vi "RTS Rebuild Custom Array.vi"(8 "Error In":errorcluster, 9 "Index Locations":i32[](array[numeric]), 10 "Full Item Names":string[](array[string]), 11 "File Location":path) -> (0 "Error Out":errorcluster, 3 "Correctly Indexed Array":dbl[][](array[numeric]))   [LabVIEW 2020]
panel:
  out "size(s) 2":i32[](array[numeric])
  out "size(s)":i32[](array[numeric])
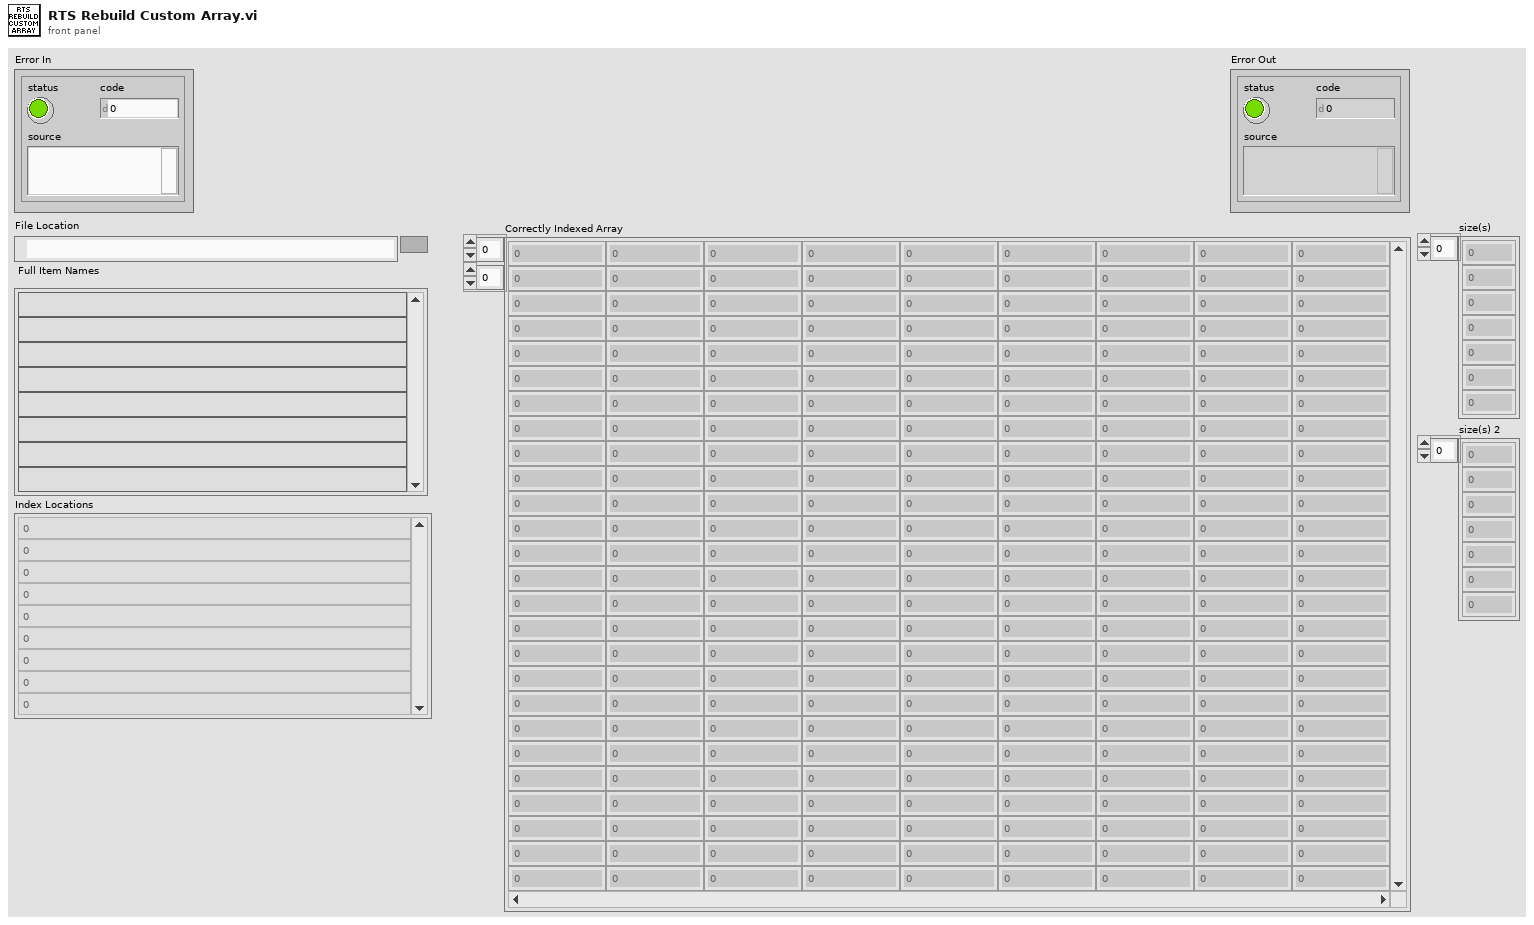
[diagram p1: front panel]
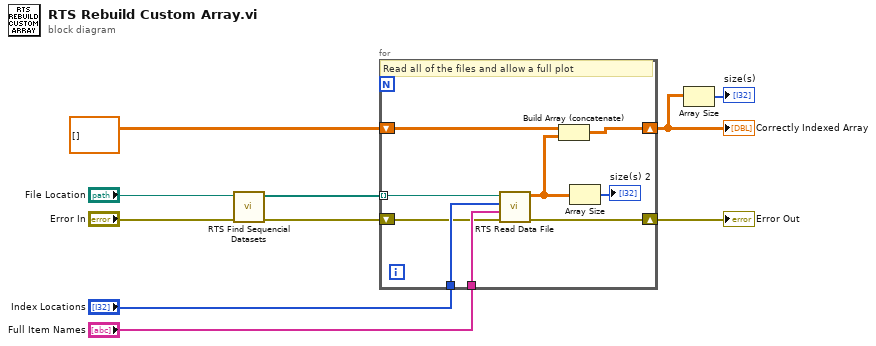
[diagram p0: block diagram]
diagram:
  n1 = call "RTS Find Sequencial Datasets.vi"("Error In"="Error In", "File Location"="File Location") -> ("Error Out"=w6:errorcluster, "Organized File Open List"=w4:path[])  [unwired: 7 in, 1 out]
  n2 = for {
    tunnel: "Full Item Names" -> [w19]
    tunnel: "Index Locations" -> [w18]
    shift-right: [w16] -> w5
    shift-left: w6 -> [w17]
    tunnel: w4 -> [w15] mode=indexing
    shift-right: [w13] -> w2
    shift-left: dbl[][] [] -> [w14]
    # "Read all of the files and allow a full plot"
    n3 = call "RTS Read Data File.vi"("Error In"=w17, "Full Item Names"=w19, "Index Locations"=w18, "File Location"=w15) -> ("Error Out"=w16:errorcluster, "Correctly Indexed Array"=w12:dbl[][])  [unwired: 6 in]
    n4 = Build Array (concatenate)(w14, w12) -> (w13:dbl[][])
    n5 = Array Size(array=w12) -> (size(s)=→"size(s) 2":i32[])
  }
  "Error Out" <- w5
  "Correctly Indexed Array" <- w2
  n6 = Array Size(array=w2) -> (size(s)=→"size(s)":i32[])
